vi "Update Points Done in Record.vi"(8 "Increment?":bool, 10 "Points Acquired":u16, 11 "Points to Acquire":u16) -> (0 "Points Done ?":bool, 2 "Points to Acquire > 0?":bool, 3 "Updated Points Acquired":u16)   [LabVIEW 2012]
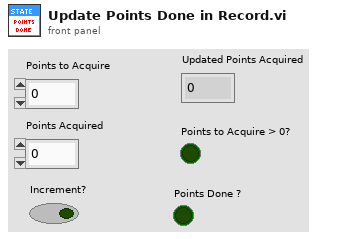
[diagram p1: front panel]
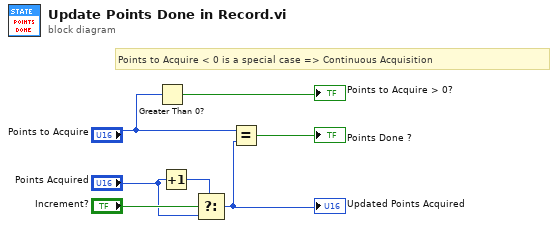
[diagram p0: block diagram]
diagram:
  # "Points to Acquire < 0 is a special case => Continuous Acquisition"
  n1 = Greater Than 0?(x="Points to Acquire") -> (x > 0?=→"Points to Acquire > 0?":bool)
  n2 = Increment(x="Points Acquired") -> (x+1=w7:u16)
  n3 = Select(t=w7, s="Increment?", f="Points Acquired") -> (s? t:f=w4:u16)
  "Updated Points Acquired" <- w4
  n4 = Equal?(x="Points to Acquire", y=w4) -> (x = y?=→"Points Done ?":bool)
